vi "Run.vi"(0 "object in":refnum<class "TowerLight.lvclass">, 5 "error in (no error)":errorcluster) -> (14 "object out":refnum<class "TowerLight.lvclass">, 19 "error out":errorcluster)   [LabVIEW 2014, in "TowerLight.lvclass"]
uses:
  TowerLight.lvclass
  TowerLight.lvclass/TowerLight.ctl
  TrafficLight.ctl
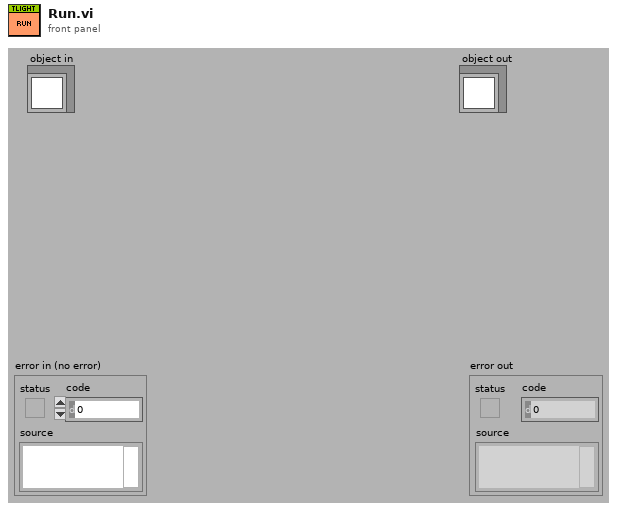
[diagram p1: front panel]
types:
  T1 = typedef "TowerLight.lvclass/TrafficLight.ctl" = cluster{"Red":bool, "Yellow":bool, "Green":bool}
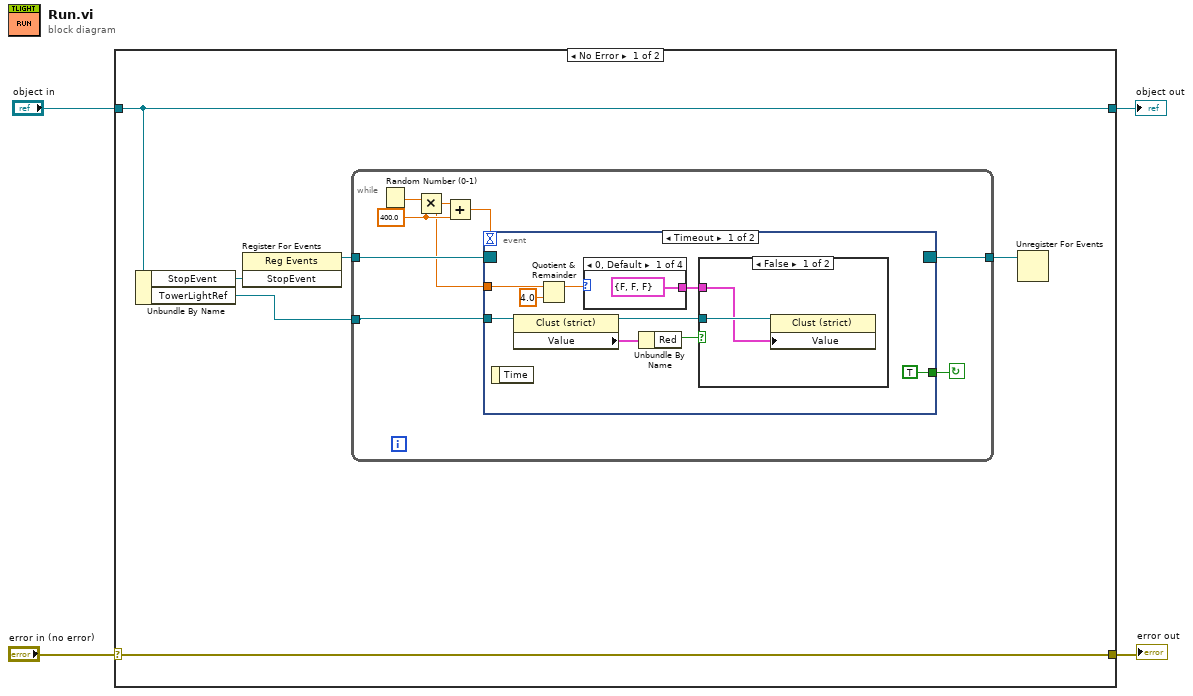
[diagram p0: block diagram]
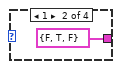
[diagram p2: hidden frame]
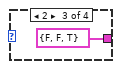
[diagram p3: hidden frame]
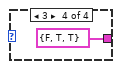
[diagram p4: hidden frame]
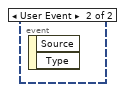
[diagram p6: hidden frame]
diagram:
  n1 = case shown="No Error" "error in (no error)" {
    selector: "error in (no error)" -> [w10 w35]
    tunnel: [w10 w35] -> w3
    tunnel: [w9 w34] -> w1
    tunnel: "object in" -> [w9 w34]
    frame No Error {
      n2 = Unbundle By Name(w9) -> ("StopEvent"=w7:refnum<user-event>, "TowerLightRef"=w6:refnum<vi>)
      n3 = register-events(w7) -> (reference out=w8:refnum<event-registration>)  [unwired: 2 in, 1 out]
      n4 = while {
        tunnel: w8 -> [w18]
        tunnel: w6 -> [w12]
        tunnel: [w11] -> w5
        stop <- w17 continue-if-true
        w16 = 400.0 ("y")
        n5 = Random Number (0-1)() -> (number: 0 to 1=w14:dbl)
        n6 = Multiply(x=w14, y=w16) -> (x*y=w13:dbl)
        n7 = Add(x=w13, y=w16) -> (x+y=w15:dbl)
        n8 = event shown="[0] Timeout" {
          selector: w18 -> [_ _]
          dyn-events: [_ _] -> w11
          timeout: w15 -> [_ _]
          tunnel: [TRUE _] -> w17
          tunnel: w13 -> [w21 _]
          tunnel: w12 -> [w26 _]
          event Timeout {
            n9 = event-data() -> ()  [unwired: 1 in, 1 out]
            n10 = property class="Clust (strict)"(reference=w26) -> (reference out=w23:refnum<vi>, "Value"=w25:T1)  [unwired: 1 in, 1 out]
            n11 = Quotient & Remainder(x=w21, y=4.0) -> (x-y*floor(x/y)=w19:dbl)  [unwired: 1 out]
            n12 = case shown="0, Default" w19 {
              tunnel: [T1 {"Red"=FALSE, "Yellow"=FALSE, "Green"=FALSE} ("Value") T1 {"Red"=FALSE, "Yellow"=TRUE, "Green"=FALSE} ("Value") T1 {"Red"=FALSE, "Yellow"=FALSE, "Green"=TRUE} ("Value") T1 {"Red"=FALSE, "Yellow"=TRUE, "Green"=TRUE} ("Value")] -> w20
              frame 0, Default {
              }
              frame 1 {
              }
              frame 2 {
              }
              frame 3 {
              }
            }
            n13 = Unbundle By Name(w25) -> ("Red"=w24:bool)
            n14 = case shown="False" w24 {
              tunnel: w23 -> [w33 _]
              tunnel: w20 -> [w32 _]
              frame False {
                n15 = property class="Clust (strict)"(reference=w33, "Value"=w32) -> ()  [unwired: 1 in, 2 out]
              }
              frame True {
              }
            }
          }
          event User Event {
            n16 = event-data() -> ()  [unwired: 1 in, 2 out]
          }
        }
      }
      n17 = Unregister For Events(event registration refnum=w5) -> ()  [unwired: 1 in, 1 out]
    }
    frame Error {
    }
  }
  "error out" <- w3
  "object out" <- w1
